vi "Save File DOE Sort Agilent List.vi"(11 "TC Channel-List":string[](array[string])) -> (2 "TC List Agilent 2":string[](array[string]), 3 "TC List Agilent 1":string[](array[string]))   [LabVIEW 2018, in "File Setup.lvlib"]
uses:
  File Setup.lvlib
  <vilib>/Utility/error.llb/whitespace.ctl
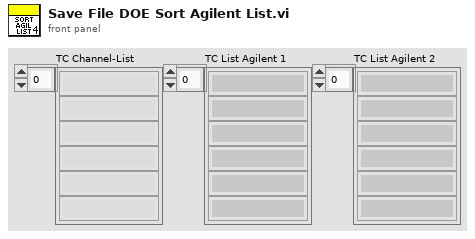
[diagram p1: front panel]
types:
  T1 = typedef "whitespace.ctl" = u16
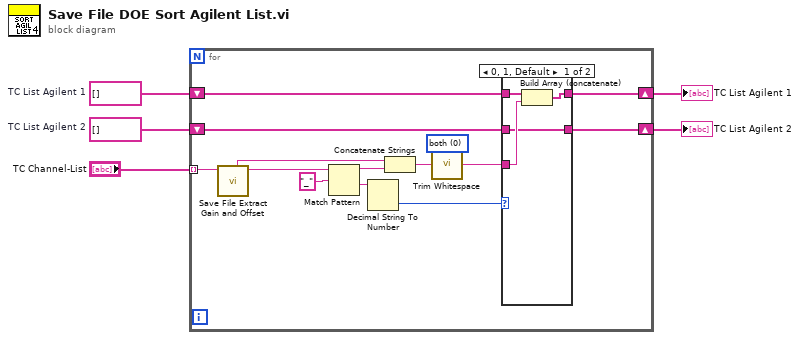
[diagram p0: block diagram]
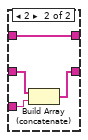
[diagram p2: hidden frame]
diagram:
  w3 = string[] []  # TC List Agilent 2
  w2 = string[] []  # TC List Agilent 1
  n1 = for {
    tunnel: "TC Channel-List" -> [w11] mode=indexing
    shift-right: [w17] -> w4
    shift-left: w2 -> [w18]
    shift-right: [w15] -> w5
    shift-left: w3 -> [w16]
    w10 = T1 0 items=["both", "start of string", "end of string"] ("location (both)")
    n2 = call "Save File Extract Gain and Offset.vi"("Analog Input"=w11) -> ("No Gain or Offset"=w9:string, "Gain & Offset"=w7:string)  [unwired: 9 in]
    n3 = Match Pattern(string=w9, regular expression="_") -> (before substring=w8:string, after substring=w13:string)  [unwired: 1 in, 2 out]
    n4 = Decimal String To Number(string=w13) -> (number=w14:i32)  [unwired: 2 in, 1 out]
    n5 = Concatenate Strings(w7, w8) -> (w6:string)
    n6 = call <vilib>:"Trim Whitespace.vi"("string"=w6, "location (both)"=w10) -> ("trimmed string"=w12:string)
    n7 = case shown="0, 1, Default" w14 {
      tunnel: w18 -> [w23 w24]
      tunnel: [w22 w24] -> w17
      tunnel: w12 -> [w21 w25]
      tunnel: w16 -> [w20 w27]
      tunnel: [w20 w26] -> w15
      frame 0, 1, Default {
        n8 = Build Array (concatenate)(w23, w21) -> (w22:string[])
      }
      frame 2 {
        n9 = Build Array (concatenate)(w27, w25) -> (w26:string[])
      }
    }
  }
  "TC List Agilent 2" <- w5
  "TC List Agilent 1" <- w4
